vi "SentinelController v35 good v11.vi"() -> ()   [LabVIEW 2011] (continued)
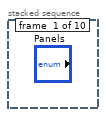
[diagram p2: hidden frame]
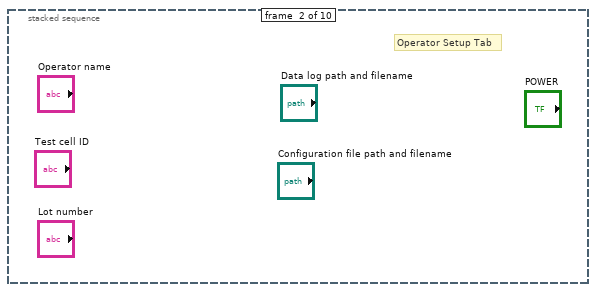
[diagram p3: hidden frame]
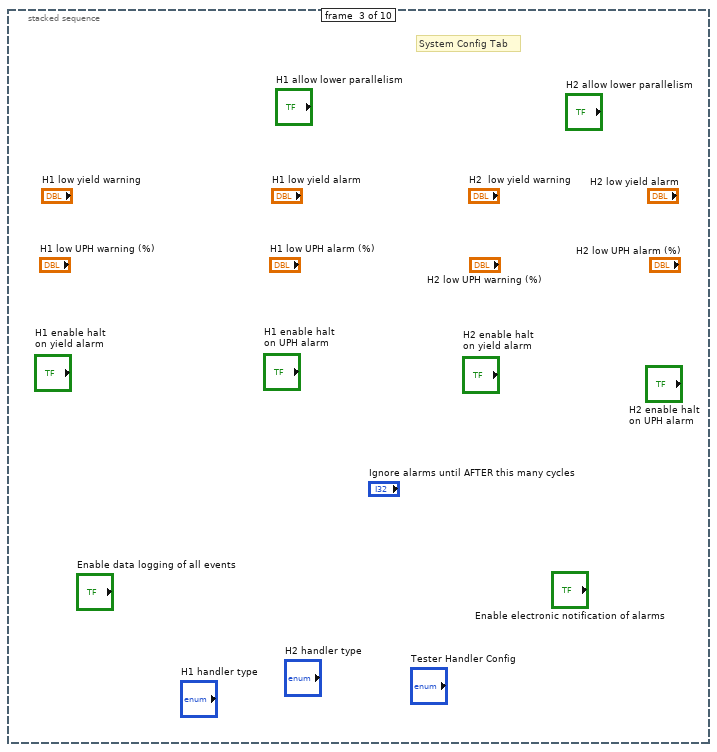
[diagram p4: hidden frame]
                                frame #0 {
                                n2576 = local read "VISA bus 2 resource name out hid"() -> (w1942:refnum<visa-resource-name>)
                                n2577 = local read "VISA bus 2 error out hid"() -> (w1941:errorcluster)
                                n2578 = VISA Close(VISA resource name=w1942, error in (no error)=w1941) -> (error out=w1940:errorcluster)
                                n2579 = Unbundle By Name(w1940) -> ("status"=w1939:bool)
                                n2580 = local write "VISA bus 2 close error"(w1939) -> ()
                                }
                                frame #1 {
                                n2581 = local write "VISA bus 2 close error"(FALSE ("VISA bus 1 close error")) -> ()
                                n2582 = Concatenate Strings("Bus 2 error  while reading,\nclosing Bus 2 and re-initializing" ("string"), "\r\n") -> (w1944:string)
                                n2583 = local write "GPIB bus 2 traffic"(w1944) -> ()
                                }
                                frame #2 {
                                n2584 = local write "MT99XX tester states H2 hid"(SC_MT99XX_tester_states."initializing bus" ("SC virtual tester states")) -> ()
                                }
                                }
                                }
                                }
                                }
                                }
                                }
                                frame "testing" {
                                n2585 = flat-sequence {
                                frame #0 {
                                n2586 = while {
                                stop <- w1948 stop-if-true
                                n2587 = local read "H2 Lock"() -> (w1948:bool)
                                n2588 = Wait (ms)(milliseconds to wait=u32 1) -> ()  [unwired: 1 out]
                                }
                                }
                                frame #1 {
                                n2589 = Tick Count (ms)() -> (millisecond timer value=w1960:u32)
                                n2590 = Tick Count (ms)() -> (millisecond timer value=w1959:u32)
                                n2591 = local write "H2 Ready with sites"(FALSE ("waiting")) -> ()
                                n2592 = local write "H2 Indexing"(FALSE ("waiting")) -> ()
                                n2593 = local write "H2 Testing"(TRUE ("testing")) -> ()
                                n2594 = local write "H2 wt end hidden"(w1960) -> ()
                                n2595 = local write "H2 tt start hidden"(w1959) -> ()
                                n2596 = local read "GPIB bus 2 traffic"() -> (w1951:string)
                                n2597 = local write "MT99XX tester states H2 hid"(SC_MT99XX_tester_states."binning" ("SC virtual tester states")) -> ()
                                n2598 = Concatenate Strings(w1951, "\r\n", "Bus 2: " ("string"), "testing" ("string")) -> (w1953:string)
                                n2599 = local write "GPIB bus 2 traffic"(w1953) -> ()
                                }
                                frame #2 {
                                n2600 = local read "H2 wt start hidden"() -> (w1962:u32)
                                n2601 = local read "H2 wt end hidden"() -> (w1961:u32)
                                n2602 = Subtract(x=w1961, y=w1962) -> (x-y=w1965:u32)
                                n2603 = Divide(x=w1965, y=u32 1000) -> (x/y=w1963:dbl)
                                n2604 = local write "H2 measured Wait Time"(w1963) -> ()
                                }
                                frame #3 {
                                n2605 = local write "MT99XX tester states H2 hid"(SC_MT99XX_tester_states."binning" ("MT99XX tester states H2 hid")) -> ()
                                }
                                }
                                }
                                frame "binning" {
                                n2606 = flat-sequence {
                                tunnel: [w1978] -> w1969
                                tunnel: [w2005] -> w1970
                                tunnel: w1969 -> [w2005]
                                tunnel: w1970 -> [w2012]
                                tunnel: [w2011] -> w1968
                                tunnel: [w2010] -> w1967
                                tunnel: w1968 -> [w2063]
                                tunnel: w1967 -> [w2062]
                                frame #0 {
                                n2607 = while {
                                stop <- w1972 continue-if-true
                                n2608 = local read "H2 Lock"() -> (w1972:bool)
                                n2609 = Wait (ms)(milliseconds to wait=u32 1) -> ()  [unwired: 1 out]
                                }
                                }
                                frame #1 {
                                n2610 = local read "Program Parallelism"() -> (w1975:u32)
                                n2611 = local read "H2 parallelism"() -> (w1974:u32)
                                n2612 = local read "H2 allow lower parallelism"() -> (w1976:bool)
                                n2613 = Less?(x=w1974, y=w1975) -> (x < y?=w1977:bool)
                                n2614 = And(x=w1977, y=w1976) -> (x .and. y?=w1973:bool)
                                n2615 = case shown="True" w1973 {
                                tunnel: [w1979 w1990] -> w1978
                                frame False {
                                n2616 = local read "VISA bus 2 resource name out hid"() -> (w1987:refnum<visa-resource-name>)
                                n2617 = local read "Binning string from tester hid"() -> (w1979:string)
                                n2618 = local read "VISA bus 2 error out hid"() -> (w1988:errorcluster)
                                n2619 = local read "GPIB bus 2 traffic"() -> (w1983:string)
                                n2620 = VISA Write(VISA resource name=w1987, write buffer=w1979, error in (no error)=w1988) -> (VISA resource name out=w1985:refnum<visa-resource-name>, error out=w1986:errorcluster)  [unwired: 1 out]
                                n2621 = local write "VISA bus 2 resource name out hid"(w1985) -> ()
                                n2622 = local write "VISA bus 2 error out hid"(w1986) -> ()
                                n2623 = Unbundle By Name(w1986) -> ("status"=w1984:bool)
                                n2624 = Concatenate Strings(w1983, "\r\n", "Bus 2 write: " ("string"), w1979) -> (w1981:string)
                                n2625 = local write "GPIB bus 2 write error"(w1984) -> ()
                                n2626 = local write "GPIB bus 2 traffic"(w1981) -> ()
                                }
                                frame True {
                                n2627 = local read "H2 parallelism"() -> (w1989:u32)
                                n2628 = local read "Binning string from tester hid"() -> (w1991:string)
                                n2629 = local read "VISA bus 2 resource name out hid"() -> (w2002:refnum<visa-resource-name>)
                                n2630 = Multiply(x=w1989, y=u32 8) -> (x*y=w1993:u32)
                                n2631 = local read "VISA bus 2 error out hid"() -> (w2003:errorcluster)
                                n2632 = local read "GPIB bus 2 traffic"() -> (w1998:string)
                                n2633 = Decrement(x=w1993) -> (x-1=w1994:u32)
                                n2634 = String Subset(string=w1991, length (rest)=w1994) -> (substring=w1990:string)  [unwired: 1 in]
                                n2635 = VISA Write(VISA resource name=w2002, write buffer=w1990, error in (no error)=w2003) -> (VISA resource name out=w2000:refnum<visa-resource-name>, error out=w2001:errorcluster)  [unwired: 1 out]
                                n2636 = local write "VISA bus 2 resource name out hid"(w2000) -> ()
                                n2637 = local write "VISA bus 2 error out hid"(w2001) -> ()
                                n2638 = Unbundle By Name(w2001) -> ("status"=w1999:bool)
                                n2639 = Concatenate Strings(w1998, "\r\n", "Bus 2 write: " ("string"), w1990) -> (w1996:string)
                                n2640 = local write "GPIB bus 2 traffic"(w1996) -> ()
                                n2641 = local write "GPIB bus 2 write error"(w1999) -> ()
                                }
                                }
                                }
                                frame #2 {
                                n2642 = Tick Count (ms)() -> (millisecond timer value=w2007:u32)
                                n2643 = Tick Count (ms)() -> (millisecond timer value=w2006:u32)
                                n2644 = local write "H2 Ready with sites"(FALSE ("waiting")) -> ()
                                n2645 = local write "H2 Testing"(FALSE ("waiting")) -> ()
                                n2646 = local write "H2 Indexing"(TRUE ("waiting")) -> ()
                                n2647 = local write "H2 it start hidden"(w2007) -> ()
                                n2648 = local write "H2 tt end hidden"(w2006) -> ()
                                }
                                frame #3 {
                                n2649 = while {
                                tunnel: [w2035] -> w2031 mode=indexing
                                shift-right: [w2036] -> _
                                shift-left: w2012 -> [w2038]
                                stop <- w2033 stop-if-true
                                n2650 = Match Pattern(string=w2038, regular expression=" ") -> (before substring=w2035:string, after substring=w2036:string, offset past match=w2034:i32)  [unwired: 2 out]
                                n2651 = Less Than 0?(x=w2034) -> (x < 0?=w2033:bool)
                                }
                                n2652 = local read "H2 tt start hidden"() -> (w2016:u32)
                                n2653 = local read "H2 tt end hidden"() -> (w2017:u32)
                                n2654 = Subtract(x=w2017, y=w2016) -> (x-y=w2015:u32)
                                n2655 = Divide(x=w2015, y=u32 1000) -> (x/y=w2013:dbl)
                                n2656 = Array Size(array=w2031) -> (size(s)=w2028:i32)
                                n2657 = local read "H2 SITES? response hid"() -> (w2023:string)
                                n2658 = local read "H2 parallelism"() -> (w2022:u32)
                                n2659 = local write "H2 measured Test Time"(w2013) -> ()
                                n2660 = Divide(x=w2028, y=3) -> (x/y=w2030:dbl)
                                n2661 = To Unsigned Byte Integer(number=w2030) -> (unsigned 8bit integer=w2026:u8)
                                n2662 = Not Equal?(x=w2022, y=w2026) -> (x != y?=w2027:bool)
                                n2663 = case shown="True" w2027 {
                                frame False {
                                }
                                frame True {
                                n2664 = One Button Dialog(message="Warning:\nH2 Parallelism Mismatch!\nEither allow this from the system configuration tab\nor change the parallelism on H2. This message will\ncontinue until the problem is corrected.") -> ()  [unwired: 1 in, 1 out]
                                }
                                }
                                n2665 = for {
                                N: w2026 -> [_]
                                tunnel: w2031 -> [w2061]
                                tunnel: w2023 -> [w2052]
                                shift-right: [w2045] -> w2010
                                shift-left: 0 -> [w2044]
                                shift-right: [w2041] -> w2011
                                shift-left: 0 -> [w2039]
                                i -> [w2042]
                                n2666 = Increment(x=w2039) -> (x+1=w2040:i32)
                                n2667 = Increment(x=w2044) -> (x+1=w2043:i32)
                                n2668 = Increment(x=w2042) -> (x+1=w2060:i32)
                                n2669 = String Subset(string=w2052, offset (0)=w2042, length (rest)=1 ("length (rest)")) -> (substring=w2048:string)
                                n2670 = Multiply(x=3, y=w2060) -> (x*y=w2054:i32)
                                n2671 = Equal?(x=w2048, y="1") -> (x = y?=w2046:bool)
                                n2672 = Select(t=w2043, s=w2046, f=w2044) -> (s? t:f=w2045:i32)
                                n2673 = Decrement(x=w2054) -> (x-1=w2053:i32)
                                n2674 = Index Array(array=w2061, index=w2053) -> (element=w2058:string)
                                n2675 = Decimal String To Number(string=w2058, offset=0) -> (number=w2056:i32)  [unwired: 1 in, 1 out]
                                n2676 = Equal?(x=w2056, y=1) -> (x = y?=w2049:bool)
                                n2677 = And(x=w2049, y=w2046) -> (x .and. y?=w2050:bool)
                                n2678 = Select(t=w2040, s=w2050, f=w2039) -> (s? t:f=w2041:i32)
                                }
                                n2679 = local read "H2 Device Count"() -> (w2019:u32)
                                n2680 = local read "H2 Good Units"() -> (w2020:u32)
                                n2681 = Add(x=w2020, y=w2011) -> (x+y=w2021:u32)
                                n2682 = Add(x=w2019, y=w2010) -> (x+y=w2018:u32)
                                n2683 = local write "H2 Good Units"(w2021) -> ()
                                n2684 = local write "H2 Device Count"(w2018) -> ()
                                }
                                frame #4 {
                                n2685 = Divide(x=w2063, y=w2062) -> (x/y=w2064:dbl)
                                n2686 = local read "H2 Device Count"() -> (w2067:u32)
                                n2687 = local read "H2 Good Units"() -> (w2068:u32)
                                n2688 = Multiply(x=w2064, y=100.0) -> (x*y=w2066:dbl)
                                n2689 = local write "H2 cycle yield hid"(w2066) -> ()
                                n2690 = Divide(x=w2068, y=w2067) -> (x/y=w2071:dbl)
                                n2691 = Multiply(x=w2071, y=100.0) -> (x*y=w2069:dbl)
                                n2692 = local write "H2 lot yield mon"(w2069) -> ()
                                }
                                frame #5 {
                                n2693 = local read "H2 online"() -> (w2072:bool)
                                n2694 = local read "POWER"() -> (w2074:bool)
                                n2695 = Compound Arithmetic op=AND(w2072, w2074) -> (w2073:bool)
                                n2696 = case shown="False" w2073 {
                                frame False {
                                n2697 = local write "MT99XX tester states H2 hid"(SC_MT99XX_tester_states."closing bus" ("SC virtual tester states")) -> ()
                                }
                                frame True {
                                n2698 = local write "MT99XX tester states H2 hid"(SC_MT99XX_tester_states."polling *SITES?" ("SC virtual tester states")) -> ()
                                }
                                }
                                }
                                }
                                }
                                frame "closing bus" {
                                n2699 = local read "GPIB bus 2 traffic"() -> (w2081:string)
                                n2700 = local write "Exit SC tester H2 StMach hid"(TRUE ("Exit H2 state machine hid")) -> ()
                                n2701 = local read "VISA bus 2 resource name out hid"() -> (w2085:refnum<visa-resource-name>)
                                n2702 = local read "VISA bus 2 error out hid"() -> (w2084:errorcluster)
                                n2703 = Concatenate Strings(w2081, "\r\n", "Bus 2: closing " ("string")) -> (w2079:string)
                                n2704 = local write "GPIB bus 2 traffic"(w2079) -> ()
                                n2705 = VISA Close(VISA resource name=w2085, error in (no error)=w2084) -> (error out=w2083:errorcluster)
                                n2706 = Unbundle By Name(w2083) -> ("status"=w2082:bool)
                                n2707 = local write "VISA bus 2 close error"(w2082) -> ()
                                }
                              }
                            }
                            frame #1 {
                              n2708 = local read "Slow for  Diagnostics"() -> (w2086:bool)
                              n2709 = case shown="True" w2086 {
                                frame False {
                                }
                                frame True {
                                n2710 = local read "GPIB wait time (ms)"() -> (w2087:u32)
                                n2711 = Wait (ms)(milliseconds to wait=w2087) -> ()  [unwired: 1 out]
                                }
                              }
                            }
                          }
                        }
                        frame "Seiko-Epson NS6040" {
                          n2712 = local write "NS6040 tester states H2 hid"(SC_NS6040_tester_states."initializing bus" ("NS6040 tester states H1 hid")) -> ()
                          n2713 = while {
                            stop <- w2089 stop-if-true
                            n2714 = flat-sequence {
                              frame #0 {
                                n2715 = local read "NS6040 tester states H2 hid"() -> (w2090:T4)
                                n2716 = case shown="\"testing\"" w2090 {
                                frame "initializing bus", Default {
                                n2717 = flat-sequence {
                                frame #0 {
                                # "bus 2"
                                n2718 = local read "GPIB wait timeout hid"() -> (w2093:u32)
                                n2719 = local read "SentCtrl talks to handler 2 at"() -> (w2095:refnum<visa-resource-name>)
                                n2720 = local read "GPIB wait timeout hid"() -> (w2094:u32)
                                n2721 = VISA Open(timeout (0)=w2093, VISA resource name=w2095) -> (VISA resource name=w2092:refnum<visa-resource-name>, error out=w2097:errorcluster)  [unwired: 3 in]
                                n2722 = property class="GPIB Instr"(reference=w2092, error in=w2097, "Timeout"=w2094) -> (error out=w2091:errorcluster)  [unwired: 1 out]
                                n2723 = local write "VISA bus 2 resource name out hid"(w2092) -> ()
                                n2724 = Unbundle By Name(w2091) -> ("status"=w2096:bool)
                                n2725 = local write "VISA bus 2 error out hid"(w2091) -> ()
                                n2726 = local write "VISA bus 2 open error"(w2096) -> ()
                                }
                                frame #1 {
                                n2727 = local write "Exit SC tester H2 StMach hid"(FALSE ("Exit H2 state machine hid")) -> ()
                                n2728 = Concatenate Strings("Bus 2 initializing" ("string"), "\r\n") -> (w2100:string)
                                n2729 = local write "GPIB bus 2 traffic"(w2100) -> ()
                                }
                                frame #2 {
                                n2730 = local write "NS6040 tester states H2 hid"(SC_NS6040_tester_states."serial polling handler" ("NS6040 tester states H2 hid")) -> ()
                                }
                                }
                                }
                                frame "sending *IDN?" {
                                n2731 = flat-sequence {
                                tunnel: [w2112] -> w2105
                                tunnel: [w2111] -> w2104
                                tunnel: w2105 -> [w2126]
                                tunnel: w2104 -> [w2125]
                                tunnel: [w2116] -> w2103
                                tunnel: w2103 -> [w2127]
                                frame #0 {
                                w2106 = "*IDN?"
                                # "It was discovered that his state is not initialized in application"
                                n2732 = local read "VISA bus 2 resource name out hid"() -> (w2115:refnum<visa-resource-name>)
                                n2733 = local read "GPIB bus 2 traffic"() -> (w2110:string)
                                n2734 = local read "VISA bus 2 error out hid"() -> (w2114:errorcluster)
                                n2735 = Concatenate Strings(w2110, "\r\n", "Bus 2 write: " ("string"), w2106) -> (w2108:string)
                                n2736 = VISA Write(VISA resource name=w2115, write buffer=w2106, error in (no error)=w2114) -> (VISA resource name out=w2112:refnum<visa-resource-name>, error out=w2111:errorcluster)  [unwired: 1 out]
                                n2737 = local write "GPIB bus 2 traffic"(w2108) -> ()
                                n2738 = Unbundle By Name(w2111) -> ("status"=w2113:bool)
                                n2739 = local write "GPIB bus 2 write error"(w2113) -> ()
                                }
                                frame #1 {
                                n2740 = VISA Read(VISA resource name=w2126, byte count=u32 256, error in (no error)=w2125) -> (VISA resource name out=w2123:refnum<visa-resource-name>, read buffer=w2117:string, error out=w2122:errorcluster)  [unwired: 1 out]
                                n2741 = local read "GPIB bus 2 traffic"() -> (w2118:string)
                                n2742 = local write "VISA bus 2 resource name out hid"(w2123) -> ()
                                n2743 = Unbundle By Name(w2122) -> ("status"=w2116:bool)
                                n2744 = local write "H2 response to *IDN? hid"(w2117) -> ()
                                n2745 = local write "GPIB bus 2 read error"(w2116) -> ()
                                n2746 = Concatenate Strings(w2118, "\r\n", "Bus 2 read: " ("string"), w2117) -> (w2120:string)
                                n2747 = local write "GPIB bus 2 traffic"(w2120) -> ()
                                }
                                frame #2 {
                                n2748 = case shown="True" w2127 {
                                frame False {
                                n2749 = local write "NS6040 tester states H2 hid"(SC_NS6040_tester_states."testing" ("NS6040 tester states H2 hid")) -> ()
                                }
                                frame True {
                                n2750 = flat-sequence {
                                frame #0 {
                                n2751 = while {
                                stop <- w2130 stop-if-true
                                n2752 = One Button Dialog(message="Warning:\nVirtual tester does not get a response\nto *IDN? from handler 2.\nCheck GPIB cable and that  handler 2 \nis running and ready to issue a start of test\nby responding with sites ready.", button name ("OK")="Dismiss and retry") -> (true=w2130:bool)
                                n2753 = Wait (ms)(milliseconds to wait=u32 100) -> ()  [unwired: 1 out]
                                }
                                }
                                frame #1 {
                                n2754 = local write "H2 online"(FALSE ("H2 online")) -> ()
                                }
                                frame #2 {
                                n2755 = local write "NS6040 tester states H2 hid"(SC_NS6040_tester_states."serial polling handler" ("NS6040 tester states H2 hid")) -> ()
                                }
                                }
                                }
                                }
                                }
                                }
                                }
                                frame "serial polling handler" {
                                w2136 = "1"
                                w2150 = "%08b"  # format string
                                n2756 = flat-sequence {
                                tunnel: [w2171] -> w2151
                                tunnel: [w2170] -> _
                                frame #0 {
                                # "This is a serial poll method that rests the SQR bits after execution"
                                n2757 = local read "GPIB bus 2 traffic"() -> (w2169:string)
                                n2758 = local read "VISA bus 2 resource name out hid"() -> (w2172:refnum<visa-resource-name>)
                                n2759 = local read "VISA bus 2 error out hid"() -> (w2173:errorcluster)
                                n2760 = Concatenate Strings(w2169, "\r\n", "Bus 2 write: " ("string"), "Serial polling handler 2") -> (w2167:string)
                                n2761 = VISA Read STB(8:w2173, 11:w2172) -> (0:w2174:errorcluster, 2:w2171:u16)  [unwired: 1 out]
                                n2762 = Unbundle By Name(w2174) -> ("status"=w2170:bool)
                                n2763 = local write "GPIB bus 2 traffic"(w2167) -> ()
                                n2764 = local write "GPIB bus 2 write error"(w2170) -> ()
                                }
                                }
                                n2765 = Format Into String "Format Into String"(format string=w2150, w2151) -> (resulting string=w2137:string)  [unwired: 2 in, 1 out]
                                n2766 = local read "GPIB bus 2 traffic"() -> (w2149:string)
                                n2767 = String Subset(string=w2137, offset (0)=1, length (rest)=1 ("length (rest)")) -> (substring=w2142:string)
                                n2768 = String Subset(string=w2137, offset (0)=7, length (rest)=1 ("length (rest)")) -> (substring=w2143:string)
                                n2769 = Equal?(x=w2142, y=w2136) -> (x = y?=w2141:bool)
                                n2770 = Equal?(x=w2136, y=w2143) -> (x = y?=w2140:bool)
                                n2771 = Concatenate Strings(w2149, "\r\n", "Bus 2 read: " ("string"), w2137) -> (w2147:string)
                                n2772 = And(x=w2141, y=w2140) -> (x .and. y?=w2135:bool)
                                n2773 = local write "GPIB bus 2 traffic"(w2147) -> ()
                                n2774 = case shown="True" w2135 {
                                frame False {
                                n2775 = flat-sequence {
                                frame #0 {
                                n2776 = Wait (ms)(milliseconds to wait=u32 5) -> ()  [unwired: 1 out]
                                }
                                frame #1 {
                                n2777 = local write "NS6040 tester states H2 hid"(SC_NS6040_tester_states."serial polling handler" ("NS6040 tester states H1 hid")) -> ()
                                }
                                }
                                }
                                frame True {
                                # "This is where the GPIB0 bus controller (PXI Chassis, instrument) has its STB set to 0100 0001 which signals to the tester that a handler is ready with sites"
                                n2778 = flat-sequence {
                                frame #0 {
                                n2779 = local write "H2 Ready with sites"(TRUE ("H2 Waiting")) -> ()
                                }
                                frame #1 {
                                n2780 = Tick Count (ms)() -> (millisecond timer value=w2158:u32)
                                n2781 = Tick Count (ms)() -> (millisecond timer value=w2157:u32)
                                n2782 = local write "H2 Indexing"(FALSE ("h1 indexing")) -> ()
                                n2783 = local write "H2 Testing"(FALSE ("h1 indexing")) -> ()
                                n2784 = local write "H2 wt start hidden"(w2158) -> ()
                                n2785 = local write "H2 it end hidden"(w2157) -> ()
                                }
                                frame #2 {
                                n2786 = local read "H2 it start hidden"() -> (w2162:u32)
                                n2787 = local read "H2 it end hidden"() -> (w2163:u32)
                                n2788 = Subtract(x=w2163, y=w2162) -> (x-y=w2159:u32)
                                n2789 = Divide(x=w2159, y=u32 1000) -> (x/y=w2161:dbl)
                                n2790 = local write "H2 measured  Index Time"(w2161) -> ()
                                }
                                frame #3 {
                                n2791 = local write "NS6040 tester states H1 hid"(SC_NS6040_tester_states."sending Fullsites?" ("NS6040 tester states H1 hid")) -> ()
                                }
                                }
                                }
                                }
                                }
                                frame "sending Fullsites?" {
                                n2792 = flat-sequence {
                                frame #0 {
                                n2793 = flat-sequence {
                                tunnel: [w2182] -> w2178
                                tunnel: [w2181] -> w2177
                                tunnel: w2178 -> [w2188]
                                tunnel: w2177 -> [w2187]
                                tunnel: [w2188] -> w2176
                                tunnel: [w2187] -> w2175
                                tunnel: w2176 -> [w2192]
                                tunnel: w2175 -> [w2191]
                                frame #0 {
                                w2179 = "FULLSITES?"
                                n2794 = local read "VISA bus 2 resource name out hid"() -> (w2183:refnum<visa-resource-name>)
                                n2795 = local read "VISA bus 2 error out hid"() -> (w2184:errorcluster)
                                n2796 = call <vilib>:"Trim Whitespace.vi"("string"=w2179) -> ("trimmed string"=w2180:string)  [unwired: 1 in]
                                n2797 = VISA Write(VISA resource name=w2183, write buffer=w2179, error in (no error)=w2184) -> (VISA resource name out=w2182:refnum<visa-resource-name>, error out=w2181:errorcluster)  [unwired: 1 out]
                                n2798 = local write "GPIB bus 2 traffic"(w2180) -> ()
                                n2799 = Unbundle By Name(w2181) -> ("status"=w2185:bool)
                                n2800 = local write "GPIB bus 2 write error"(w2185) -> ()
                                }
                                frame #1 {
                                n2801 = Wait (ms)(milliseconds to wait=u32 2) -> ()  [unwired: 1 out]
                                }
                                frame #2 {
                                n2802 = local read "GPIB bus 2 traffic"() -> (w2199:string)
                                n2803 = VISA Read(VISA resource name=w2192, byte count=u32 256, error in (no error)=w2191) -> (VISA resource name out=w2197:refnum<visa-resource-name>, read buffer=w2189:string, error out=w2194:errorcluster)  [unwired: 1 out]
                                n2804 = local write "H2 FULLSITES? response hid"(w2189) -> ()
                                n2805 = Unbundle By Name(w2194) -> ("status"=w2200:bool)
                                n2806 = local write "VISA bus 2 resource name out hid"(w2197) -> ()
                                n2807 = call <vilib>:"Trim Whitespace.vi"("string"=w2189) -> ("trimmed string"=w2190:string)  [unwired: 1 in]
                                n2808 = local write "GPIB bus 2 read error"(w2200) -> ()
                                n2809 = Concatenate Strings(w2199, "\r\n", "Bus 2 read: " ("string"), w2190) -> (w2198:string)
                                n2810 = local write "GPIB bus 2 traffic"(w2198) -> ()
                                }
                                }
                                }
                                frame #1 {
                                n2811 = local read "GPIB bus 2 read error"() -> (w2201:bool)
                                n2812 = case shown="False" w2201 {
                                frame False {
                                n2813 = flat-sequence {
                                frame #0 {
                                w2210 = "%032b"  # format string
                                n2814 = local read "H2 FULLSITES? response hid"() -> (w2203:string)
                                n2815 = call <vilib>:"Space Constant.vi"() -> ("String"=w2205:string)
                                n2816 = Concatenate Strings("Fullsites?\n" ("regular expression"), w2205) -> (w2204:string)
                                n2817 = call <vilib>:"Trim Whitespace.vi"("string"=w2203) -> ("trimmed string"=w2202:string)  [unwired: 1 in]
                                n2818 = Match Pattern(string=w2202, regular expression=w2204) -> (after substring=w2208:string)  [unwired: 1 in, 3 out]
                                n2819 = Hexadecimal String To Number(string=w2208, default (0uL)=u64 0 ("default (0 U32)")) -> (number=w2211:u64)  [unwired: 1 in, 1 out]
                                n2820 = Format Into String "Format Into String"(format string=w2210, w2211) -> (resulting string=w2207:string)  [unwired: 2 in, 1 out]
                                n2821 = local write "H2 FULLSITES? binary hid"(w2207) -> ()
                                }
                                frame #1 {
                                n2822 = while {
                                stop <- w2212 stop-if-true
                                n2823 = local read "H2 Lock"() -> (w2212:bool)
                                n2824 = Wait (ms)(milliseconds to wait=u32 1) -> ()  [unwired: 1 out]
                                }
                                }
                                frame #2 {
                                n2825 = local write "NS6040 tester states H2 hid"(SC_NS6040_tester_states."testing" ("NS6040 tester states H1 hid")) -> ()
                                }
                                }
                                }
                                frame True {
                                n2826 = flat-sequence {
                                frame #0 {
                                n2827 = while {
                                stop <- w2215 stop-if-true
                                n2828 = Wait (ms)(milliseconds to wait=u32 100) -> ()  [unwired: 1 out]
                                n2829 = One Button Dialog(message="Read error while reading FULLSITES?,\nclosing Bus and re-initializing" ("Reply from Sentinel Controller to tester")) -> (true=w2215:bool)  [unwired: 1 in]
                                }
                                }
                                frame #1 {
                                n2830 = local read "VISA bus 2 resource name out hid"() -> (w2218:refnum<visa-resource-name>)
                                n2831 = local read "VISA bus 2 error out hid"() -> (w2219:errorcluster)
                                n2832 = VISA Close(VISA resource name=w2218, error in (no error)=w2219) -> (error out=w2221:errorcluster)
                                n2833 = Unbundle By Name(w2221) -> ("status"=w2220:bool)
                                n2834 = local write "VISA bus 2 close error"(w2220) -> ()
                                }
                                frame #2 {
                                n2835 = local write "VISA bus 2 close error"(FALSE ("H1 online")) -> ()
                                n2836 = local write "NS6040 tester states H2 hid"(SC_NS6040_tester_states."initializing bus" ("NS6040 tester states H1 hid")) -> ()
                                }
                                }
                                }
                                }
                                }
                                }
                                }
                                frame "testing" {
                                n2837 = flat-sequence {
                                frame #0 {
                                n2838 = local read "GPIB bus 2 traffic"() -> (w2227:string)
                                n2839 = Concatenate Strings(w2227, "\r\n", "Bus 2: " ("string"), "testing" ("string")) -> (w2225:string)
                                n2840 = local write "GPIB bus 2 traffic"(w2225) -> ()
                                }
                                frame #1 {
                                n2841 = Tick Count (ms)() -> (millisecond timer value=w2232:u32)
                                n2842 = Tick Count (ms)() -> (millisecond timer value=w2233:u32)
                                n2843 = local write "H2 Indexing"(FALSE ("waiting")) -> ()
                                n2844 = local write "H2 Testing"(TRUE ("testing")) -> ()
                                n2845 = local write "H2 Ready with sites"(FALSE ("waiting")) -> ()
                                n2846 = local write "H2 tt start hidden"(w2232) -> ()
                                n2847 = local write "H2 wt end hidden"(w2233) -> ()
                                }
                                frame #2 {
                                n2848 = local read "H2 wt start hidden"() -> (w2235:u32)
                                n2849 = local read "H2 wt end hidden"() -> (w2234:u32)
                                n2850 = Subtract(x=w2234, y=w2235) -> (x-y=w2238:u32)
                                n2851 = Divide(x=w2238, y=u32 1000) -> (x/y=w2236:dbl)
                                n2852 = local write "H2 measured Wait Time"(w2236) -> ()
                                }
                                frame #3 {
                                n2853 = while {
                                stop <- w2240 continue-if-true
                                n2854 = local read "H2 Lock"() -> (w2240:bool)
                                n2855 = Wait (ms)(milliseconds to wait=u32 1) -> ()  [unwired: 1 out]
                                }
                                }
                                frame #4 {
                                n2856 = local write "NS6040 tester states H2 hid"(SC_NS6040_tester_states."sending BINON?" ("NS6040 tester states H1 hid")) -> ()
                                }
                                }
                                }
                                frame "sending BINON?" {
                                n2857 = flat-sequence {
                                tunnel: [w2252] -> w2243
                                tunnel: [w2251] -> w2242
                                tunnel: w2243 -> [w2261]
                                tunnel: w2242 -> [w2260]
                                frame #0 {
                                n2858 = while {
                                stop <- w2245 stop-if-true
                                n2859 = local read "Binning string from tester hid"() -> (w2246:string)
                                n2860 = Wait (ms)(milliseconds to wait=u32 5) -> ()  [unwired: 1 out]
                                n2861 = String Length(string=w2246) -> (length=w2247:i32)
                                n2862 = Greater Than 0?(x=w2247) -> (x > 0?=w2245:bool)
                                }
                                }
                                frame #1 {
                                n2863 = local write "H2 Ready with sites"(FALSE ("waiting")) -> ()
                                }
                                frame #2 {
                                n2864 = local read "VISA bus 2 resource name out hid"() -> (w2258:refnum<visa-resource-name>)
                                n2865 = local read "Binning string from tester hid"() -> (w2249:string)
                                n2866 = local read "VISA bus 2 error out hid"() -> (w2259:errorcluster)
                                n2867 = local read "GPIB bus 2 traffic"() -> (w2256:string)
                                n2868 = VISA Write(VISA resource name=w2258, write buffer=w2249, error in (no error)=w2259) -> (VISA resource name out=w2252:refnum<visa-resource-name>, error out=w2251:errorcluster)  [unwired: 1 out]
                                n2869 = local write "VISA bus 2 error out hid"(w2251) -> ()
                                n2870 = Unbundle By Name(w2251) -> ("status"=w2257:bool)
                                n2871 = call <vilib>:"Trim Whitespace.vi"("string"=w2249) -> ("trimmed string"=w2250:string)  [unwired: 1 in]
                                n2872 = local write "GPIB bus 2 write error"(w2257) -> ()
                                n2873 = Concatenate Strings(w2256, "\r\n", "Bus 2 write: " ("string"), w2250) -> (w2254:string)
                                n2874 = local write "GPIB bus 2 traffic"(w2254) -> ()
                                }
                                frame #3 {
                                n2875 = while {
                                tunnel: w2261 -> [w2268]
                                tunnel: w2260 -> [w2267]
                                stop <- w2264 stop-if-true
                                n2876 = local read "GPIB bus 2 traffic"() -> (w2270:string)
                                n2877 = VISA Read(VISA resource name=w2268, byte count=u32 256, error in (no error)=w2267) -> (VISA resource name out=w2275:refnum<visa-resource-name>, read buffer=w2262:string, error out=w2274:errorcluster)  [unwired: 1 out]
                                n2878 = local write "VISA bus 2 resource name out hid"(w2275) -> ()
                                n2879 = Unbundle By Name(w2274) -> ("status"=w2269:bool)
                                n2880 = Match True/False String(2:"false string" ("false string"), 3:"ECHO:", 4:w2262) -> (0:w2264:bool)  [unwired: 1 out]
                                n2881 = local write "GPIB bus 2 read error"(w2269) -> ()
                                n2882 = call <vilib>:"Trim Whitespace.vi"("string"=w2262) -> ("trimmed string"=w2263:string)  [unwired: 1 in]
                                n2883 = Concatenate Strings(w2270, "\r\n", "Bus 2 read: " ("string"), w2263) -> (w2272:string)
                                n2884 = local write "H2 echo hid"(w2262) -> ()
                                n2885 = local write "GPIB bus 2 traffic"(w2272) -> ()
                                }
                                }
                                frame #4 {
                                n2886 = while {
                                stop <- w2277 continue-if-true
                                n2887 = local read "Echo state of tester hid"() -> (w2279:T3)
                                n2888 = Equal?(x=w2279, y=Echo_tester_states."NO ECHO") -> (x = y?=w2277:bool)
                                n2889 = Wait (ms)(milliseconds to wait=u32 5) -> ()  [unwired: 1 out]
                                }
                                }
                                frame #5 {
                                n2890 = local read "GPIB bus 2 read error"() -> (w2281:bool)
                                n2891 = case shown="False" w2281 {
                                frame False {
                                n2892 = local read "Echo state of tester hid"() -> (w2282:T3)
                                n2893 = case shown="\"ECHONG\", Default" w2282 {
                                frame "ECHONG", Default {
                                n2894 = local write "NS6040 tester states H2 hid"(SC_NS6040_tester_states."sending ECHONG" ("NS6040 tester states H2 hid")) -> ()
                                }
                                frame "ECHOOK" {
                                n2895 = local write "NS6040 tester states H2 hid"(SC_NS6040_tester_states."sending ECHOOK" ("NS6040 tester states H2 hid")) -> ()
                                }
                                }
                                }
                                frame True {
                                n2896 = flat-sequence {
                                frame #0 {
                                n2897 = while {
                                stop <- w2286 stop-if-true
                                n2898 = Wait (ms)(milliseconds to wait=u32 100) -> ()  [unwired: 1 out]
                                n2899 = One Button Dialog(message="Echo readback error for H2.\nClosing Bus 2.", button name ("OK")="Dismiss") -> (true=w2286:bool)
                                }
                                }
                                frame #1 {
                                n2900 = local write "NS6040 tester states H2 hid"(SC_NS6040_tester_states."closing bus" ("NS6040 tester states H1 hid")) -> ()
                                }
                                }
                                }
                                }
                                }
                                }
                                }
                                frame "sending ECHONG" {
                                n2901 = flat-sequence {
                                frame #0 {
                                w2290 = "ECHONG\n"
                                n2902 = local read "VISA bus 2 resource name out hid"() -> (w2298:refnum<visa-resource-name>)
                                n2903 = local read "VISA bus 2 error out hid"() -> (w2299:errorcluster)
                                n2904 = local read "GPIB bus 2 traffic"() -> (w2296:string)
                                n2905 = VISA Write(VISA resource name=w2298, write buffer=w2290, error in (no error)=w2299) -> (error out=w2292:errorcluster)  [unwired: 2 out]
                                n2906 = local write "VISA bus 2 error out hid"(w2292) -> ()
                                n2907 = Unbundle By Name(w2292) -> ("status"=w2297:bool)
                                n2908 = call <vilib>:"Trim Whitespace.vi"("string"=w2290) -> ("trimmed string"=w2291:string)  [unwired: 1 in]
                                n2909 = local write "GPIB bus 2 write error"(w2297) -> ()
                                n2910 = Concatenate Strings(w2296, "\r\n", "Bus 2 write: " ("string"), w2291) -> (w2294:string)
                                n2911 = local write "GPIB bus 2 traffic"(w2294) -> ()
                                }
                                frame #1 {
                                n2912 = while {
                                stop <- w2300 stop-if-true
                                n2913 = Wait (ms)(milliseconds to wait=u32 100) -> ()  [unwired: 1 out]
                                n2914 = One Button Dialog(message="ECHO from handler 2 did not match BINON'\nError message from \"sending ECHONG\" state\nBINON message will be resent.") -> (true=w2300:bool)  [unwired: 1 in]
                                }
                                }
                                frame #2 {
                                n2915 = local write "NS6040 tester states H2 hid"(SC_NS6040_tester_states."sending BINON?" ("NS6040 tester states H1 hid")) -> ()
                                }
                                }
                                }
                                frame "sending ECHOOK" {
                                n2916 = flat-sequence {
                                frame #0 {
                                w2304 = "ECHOOK\n"
                                n2917 = local read "VISA bus 2 resource name out hid"() -> (w2312:refnum<visa-resource-name>)
                                n2918 = local read "VISA bus 2 error out hid"() -> (w2313:errorcluster)
                                n2919 = local read "GPIB bus 2 traffic"() -> (w2310:string)
                                n2920 = VISA Write(VISA resource name=w2312, write buffer=w2304, error in (no error)=w2313) -> (error out=w2306:errorcluster)  [unwired: 2 out]
                                n2921 = local write "VISA bus 2 error out hid"(w2306) -> ()
                                n2922 = Unbundle By Name(w2306) -> ("status"=w2311:bool)
                                n2923 = call <vilib>:"Trim Whitespace.vi"("string"=w2304) -> ("trimmed string"=w2305:string)  [unwired: 1 in]
                                n2924 = local write "GPIB bus 2 write error"(w2311) -> ()
                                n2925 = Concatenate Strings(w2310, "\r\n", "Bus 2 write: " ("string"), w2305) -> (w2308:string)
                                n2926 = local write "GPIB bus 2 traffic"(w2308) -> ()
                                }
                                frame #1 {
                                n2927 = Tick Count (ms)() -> (millisecond timer value=w2315:u32)
                                n2928 = Tick Count (ms)() -> (millisecond timer value=w2316:u32)
                                n2929 = local write "H2 Ready with sites"(FALSE ("waiting")) -> ()
                                n2930 = local write "H2 Testing"(FALSE ("waiting")) -> ()
                                n2931 = local write "H2 Indexing"(TRUE ("waiting")) -> ()
                                n2932 = local write "H2 tt end hidden"(w2315) -> ()
                                n2933 = local write "H2 it start hidden"(w2316) -> ()
                                }
                                frame #2 {
                                n2934 = local read "H2 tt start hidden"() -> (w2322:u32)
                                n2935 = local read "H2 tt end hidden"() -> (w2323:u32)
                                n2936 = Subtract(x=w2323, y=w2322) -> (x-y=w2321:u32)
                                n2937 = Divide(x=w2321, y=u32 1000) -> (x/y=w2319:dbl)
                                n2938 = local write "H2 measured Test Time"(w2319) -> ()
                                }
                                frame #3 {
                                n2939 = local read "H2 binning string hid"() -> (w2324:string)
                                n2940 = local read "H2 FULLSITES? binary hid"() -> (w2341:string)
                                n2941 = String Subset(string=w2324, offset (0)=6, length (rest)=35 ("length (rest)")) -> (substring=w2338:string)
                                n2942 = local read "H2 Device Count"() -> (w2326:u32)
                                n2943 = local read "H2 Good Units"() -> (w2328:u32)
                                n2944 = Search and Replace String(replace all?=TRUE ("replace all? (F)"), input string=w2338, search string=",") -> (result string=w2332:string)  [unwired: 5 in, 3 out]
                                n2945 = Search and Replace String(replace all?=TRUE ("replace all? (F)"), input string=w2341, search string="1") -> (number of replacements=w2342:i32)  [unwired: 5 in, 3 out]
                                n2946 = Add(x=w2342, y=w2326) -> (x+y=w2325:u32)
                                n2947 = Divide(x=w2328, y=w2326) -> (x/y=w2331:dbl)
                                n2948 = Search and Replace String(replace all?=TRUE ("replace all? (F)"), input string=w2332, search string="1") -> (number of replacements=w2333:i32)  [unwired: 5 in, 3 out]
                                n2949 = local write "H2 Device Count"(w2325) -> ()
                                n2950 = Add(x=w2333, y=w2328) -> (x+y=w2327:u32)
                                n2951 = Multiply(x=w2331, y=100.0) -> (x*y=w2329:dbl)
                                n2952 = local write "H2 Good Units"(w2327) -> ()
                                n2953 = local write "H2 cycle yield hid"(w2329) -> ()
                                }
                                frame #4 {
                                n2954 = local read "H2 Device Count"() -> (w2345:u32)
                                n2955 = local read "H2 Good Units"() -> (w2346:u32)
                                n2956 = Divide(x=w2346, y=w2345) -> (x/y=w2349:dbl)
                                n2957 = Multiply(x=w2349, y=100.0) -> (x*y=w2347:dbl)
                                n2958 = local write "H2 lot yield mon"(w2347) -> ()
                                }
                                frame #5 {
                                n2959 = local read "H2 online"() -> (w2350:bool)
                                n2960 = local read "POWER"() -> (w2352:bool)
                                n2961 = Compound Arithmetic op=AND(w2350, w2352) -> (w2351:bool)
                                n2962 = case shown="False" w2351 {
                                frame False {
                                n2963 = local write "NS6040 tester states H2 hid"(SC_NS6040_tester_states."closing bus" ("NS6040 tester states H2 hid")) -> ()
                                }
                                frame True {
                                n2964 = local write "NS6040 tester states H2 hid"(SC_NS6040_tester_states."serial polling handler" ("NS6040 tester states H2 hid")) -> ()
                                }
                                }
                                }
                                }
                                }
                                frame "closing bus" {
                                n2965 = local read "GPIB bus 2 traffic"() -> (w2359:string)
                                n2966 = local write "Exit SC tester H2 StMach hid"(TRUE ("Exit H2 state machine hid")) -> ()
                                n2967 = local read "VISA bus 2 resource name out hid"() -> (w2363:refnum<visa-resource-name>)
                                n2968 = local read "VISA bus 2 error out hid"() -> (w2362:errorcluster)
                                n2969 = Concatenate Strings(w2359, "\r\n", "Bus 2: closing " ("string")) -> (w2357:string)
                                n2970 = local write "GPIB bus 2 traffic"(w2357) -> ()
                                n2971 = VISA Close(VISA resource name=w2363, error in (no error)=w2362) -> (error out=w2361:errorcluster)
                                n2972 = Unbundle By Name(w2361) -> ("status"=w2360:bool)
                                n2973 = local write "VISA bus 2 close error"(w2360) -> ()
                                }
                                }
                              }
                              frame #1 {
                                n2974 = local read "Slow for  Diagnostics"() -> (w2364:bool)
                                n2975 = case shown="True" w2364 {
                                frame False {
                                }
                                frame True {
                                n2976 = local read "GPIB wait time (ms)"() -> (w2365:u32)
                                n2977 = Wait (ms)(milliseconds to wait=w2365) -> ()  [unwired: 1 out]
                                }
                                }
                              }
                            }
                            n2978 = local read "Exit SC tester H2 StMach hid"() -> (w2089:bool)
                          }
                        }
                      }
                    }
                  }
                }
              }
              n2979 = local read "POWER"() -> (w1814:bool)
            }
          }
        }
      }
    }
  }
